vi "Update Values from JSON.vi"(0 "JSON String":string, 5 "VI Ref In":refnum<vi>, 11 "Error In":errorcluster) -> (4 "VI Ref Out":refnum<vi>, 15 "Error Out":errorcluster)   [LabVIEW 2019, in "SLL JSON to Cluster.lvlib"]
doc: "This VI updates JSON values into the created cluster"
uses:
  SLL JSON to Cluster.lvlib
  <vilib>/Utility/miscctls.llb/LVPositionTypeDef.ctl
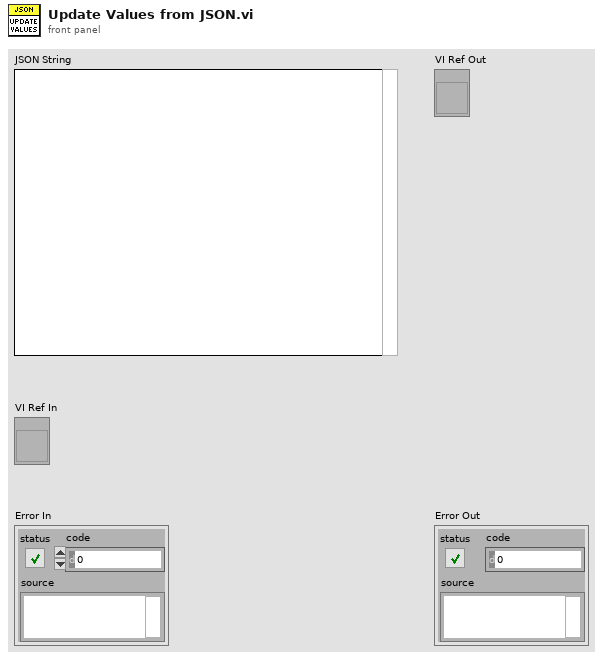
[diagram p1: front panel]
types:
  T1 = typedef "LVPositionTypeDef.ctl" = cluster{"Left":i32, "Top":i32}
  T2 = typedef "SLL JSON to Cluster.lvlib/Control Terminal Reference.ctl" = cluster{"Terminal":refnum<vi>, "Control Label":string}
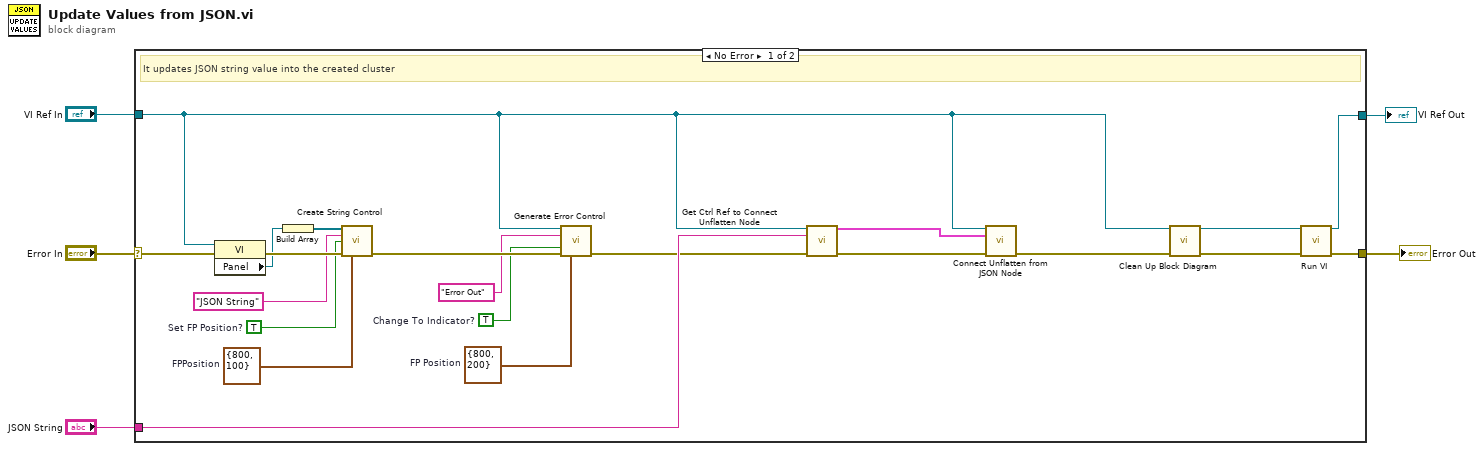
[diagram p0: block diagram]
diagram:
  n1 = case shown="No Error" "Error In" {
    selector: "Error In" -> [w20 w27]
    tunnel: [w25 w27] -> w5
    tunnel: "JSON String" -> [w24 _]
    tunnel: "VI Ref In" -> [w8 w28]
    tunnel: [w6 w28] -> w1
    frame No Error {
      w14 = T1 {"Left"=800, "Top"=100}  # FPPosition
      w9 = T1 {"Left"=800, "Top"=200}  # FP Position
      w10 = TRUE  # Change To Indicator?
      w15 = TRUE  # Set FP Position?
      # "It updates JSON string value into the created cluster"
      n2 = property class="VI"(reference=w8, error in=w20) -> (error out=w19:errorcluster, "Panel"=w18:refnum<vi>)  [unwired: 1 out]
      n3 = Build Array(w18) -> (w17:refnum<vi>[])
      n4 = call "Create String Control.vi"("Parent Ref In"=w17, "String Control label"="JSON String" ("Label.Text"), "Set FP Position"=w15, "Error In"=w19, "Position"=w14) -> ("Error Out"=w13:errorcluster)  [unwired: 10 in]
      n5 = call "Generate Error Control.vi"("VI Ref In"=w8, "Label"="Error Out", "Change To Indicator?"=w10, "Error In"=w13, "FP Position"=w9) -> ("Error Out"=w12:errorcluster)  [unwired: 10 in]
      n6 = call "Get Ctrl Ref to Connect Unflatten Node.vi"("VI Ref In"=w8, "JSON String"=w24, "Error In"=w12) -> ("Control Terminal References"=w7:T2[], "Error Out"=w26:errorcluster)  [unwired: 11 in]
      n7 = call "Connect Unflatten from JSON Node.vi"("VI Ref In"=w8, "Control Terminal References"=w7, "Error In"=w26) -> ("Error Out"=w23:errorcluster)  [unwired: 12 in]
      n8 = call "Clean Up Block Diagram.vi"("VI Ref In"=w8, "Error In"=w23) -> ("VI Ref Out"=w21:refnum<vi>, "Error Out"=w22:errorcluster)  [unwired: 12 in]
      n9 = call "Run VI.vi"("VI Ref In"=w21, "Error In"=w22) -> ("VI Ref Out"=w6:refnum<vi>, "Error Out"=w25:errorcluster)  [unwired: 12 in]
    }
    frame Error {
      # "If error, this case pass that error message only"
    }
  }
  "Error Out" <- w5
  "VI Ref Out" <- w1
